vi "Scan Mode Panel.vi"(8 "error in (no error)":errorcluster, 11 "Scan SBlock in":refnum<class "Scan SBlock.lvclass">) -> (0 "error out":errorcluster, 2 "Parameters out":string[][][](array[string]), 3 "Schedule Block out":refnum<class "Schedule Block.lvclass">)   [LabVIEW 2020, in "TALOS.lvlib" / "Run Utilities.lvlib" / "Scan SBlock.lvclass"]
uses:
  Scan SBlock.lvclass
  Advanced Parameters.ctl
  Advanced Panel Parameter Mode.ctl
  Advanced Parameters - list.ctl
  Schedule Block/Schedule Block.lvclass
  C:/LabVIEW Code/TALOS/talos/Run Utilities/Schedule Block/Schedule Block.lvclass
panel:
  in  "Array from List":T1[](array[typedef]) caption="Parameters"
  in  "No. of steps":u32
  in  "Array of Parameters":T2[](array[typedef])
  # "Parameter"
  # "Values"
  # "If the LINKED mode is used the Step size is ignored, and it is calculated based on the number of steps -->"
  # "Parameter"
  # "From"
  # "To"
  # "Step"
  # "Mode"
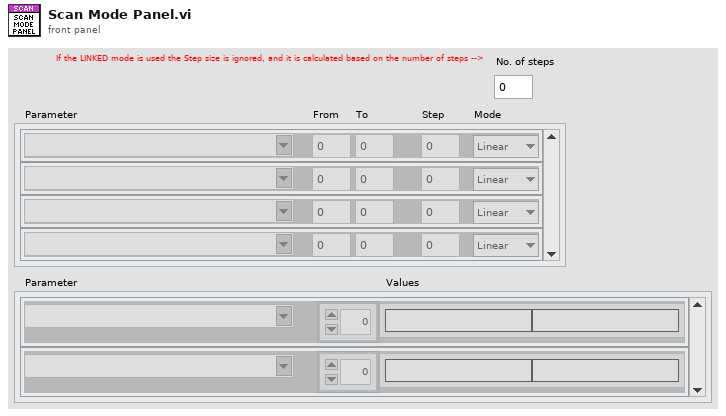
[diagram p1: front panel]
types:
  T1 = typedef "TALOS.lvlib/Run Utilities.lvlib/Scan SBlock.lvclass/Advanced Parameters - list.ctl" = cluster{"Param":string, "List of values":string[]}
  T2 = typedef "TALOS.lvlib/Run Utilities.lvlib/Scan SBlock.lvclass/Advanced Parameters.ctl" = cluster{"Param":string, "From":dbl, "To":dbl, "Step":dbl, "Mode":T3}
  T3 = typedef "TALOS.lvlib/Run Utilities.lvlib/Scan SBlock.lvclass/Advanced Panel Parameter Mode.ctl" = enum16{"Linear", "Log", "LINKED"}
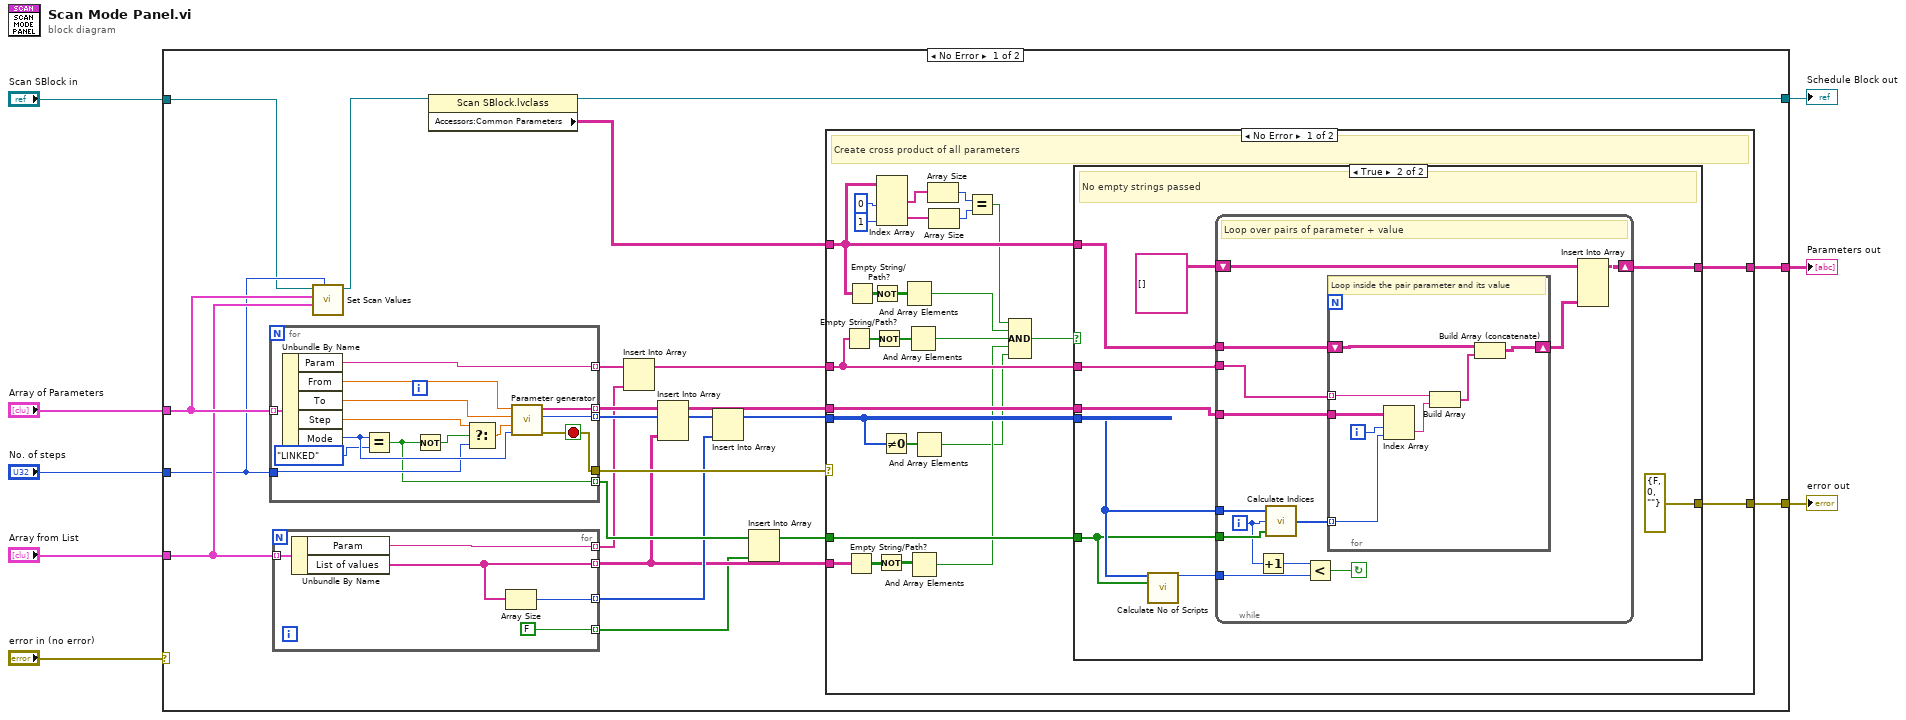
[diagram p0: block diagram]
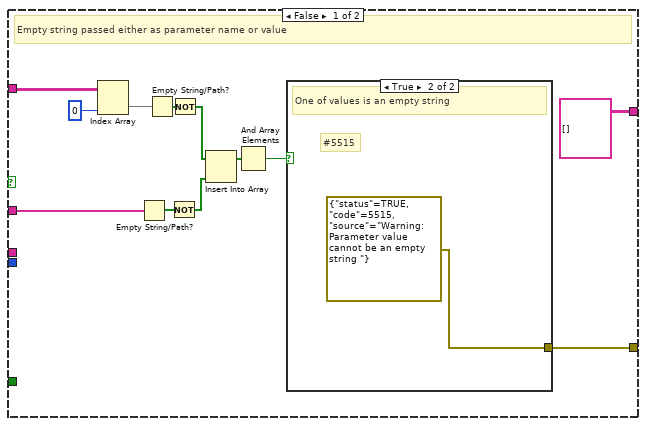
[diagram p2: hidden frame]
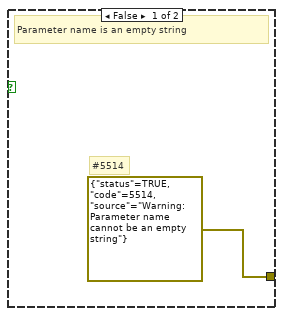
[diagram p3: hidden frame]
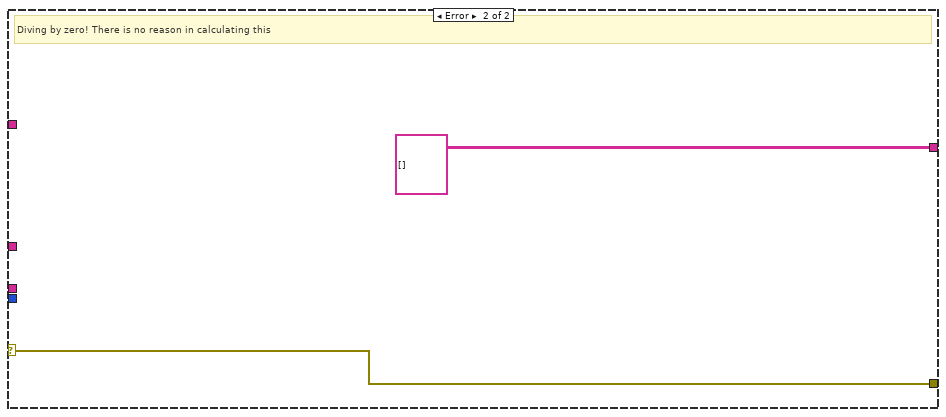
[diagram p4: hidden frame]
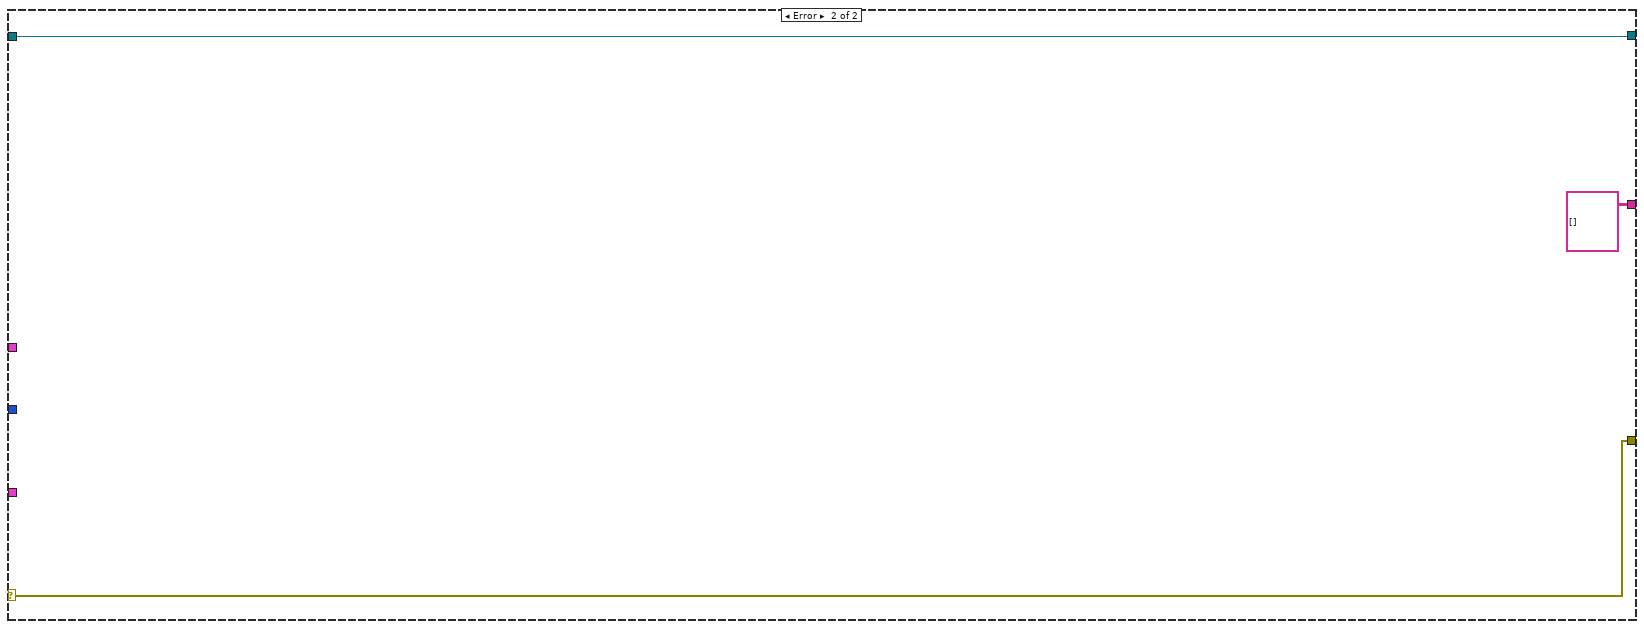
[diagram p5: hidden frame]
diagram:
  n1 = case shown="No Error" "error in (no error)" {
    selector: "error in (no error)" -> [_ w124]
    tunnel: [w29 string[][][] [] ("Parameters out")] -> w8
    tunnel: [w28 w124] -> w7
    tunnel: "Array of Parameters" -> [w15 _]
    tunnel: "Array from List" -> [w14 _]
    tunnel: "No. of steps" -> [w13 _]
    tunnel: "Scan SBlock in" -> [w12 w125]
    tunnel: [w9 w125] -> w2
    frame No Error {
      n2 = for {
        tunnel: w15 -> [w46] mode=indexing
        tunnel: w13 -> [w44]
        tunnel: [w42] -> w30
        tunnel: [w45] -> w24 mode=indexing
        tunnel: [w36] -> w26 mode=indexing
        tunnel: [w41] -> w27 mode=indexing
        tunnel: [w39] -> w25 mode=indexing
        stop <- w42 stop-if-true
        n3 = Unbundle By Name(w46) -> ("Param"=w45:string, "From"=w43:dbl, "To"=w47:dbl, "Step"=w48:dbl, "Mode"=w49:T3)
        n4 = Equal?(x=w49, y=Advanced_Panel_Parameter_Mode."LINKED") -> (x = y?=w36:bool)
        n5 = Not(x=w36) -> (.not. x?=w37:bool)
        n6 = Select(t=w48, s=w37, f=w44) -> (s? t:f=w40:dbl)
        n7 = call "Parameter generator.vi"("Mode"=w49, "Step/Iterations"=w40, "To"=w47, "From"=w43) -> ("error out"=w42:errorcluster, "Size of the array"=w41:i32, "Array of parameter values"=w39:string[])  [unwired: 5 in]
      }
      n8 = for {
        tunnel: w14 -> [w35] mode=indexing
        tunnel: [w34] -> w19 mode=indexing
        tunnel: [w33] -> w22 mode=indexing
        tunnel: [w32] -> w17 mode=indexing
        tunnel: [FALSE] -> w16 mode=indexing
        n9 = Unbundle By Name(w35) -> ("Param"=w33:string, "List of values"=w32:string[])
        n10 = Array Size(array=w32) -> (size(s)=w34:i32)
      }
      n11 = call-dynamic "Set Scan Values.vi"("No. of steps"=w13, "Array from List"=w14, "Array of Parameters"=w15, "Scan SBlock in"=w12) -> ("Scan SBlock out"=w10:refnum<class "Scan SBlock.lvclass">)  [unwired: 6 in, 1 out]
      n12 = property class="Scan SBlock.lvclass"(reference=w10) -> (reference out=w9:refnum<class "Scan SBlock.lvclass">, "Accessors:Common Parameters"=w11:string[][])  [unwired: 1 in, 1 out]
      n13 = Insert Into Array(array=w24, new element=w22) -> (w23:string[])  [unwired: 1 in]
      n14 = Insert Into Array(array=w25, new element=w17) -> (w21:string[][])  [unwired: 2 in]
      n15 = Insert Into Array(array=w27, new element=w19) -> (w20:i32[])  [unwired: 1 in]
      n16 = Insert Into Array(array=w26, new element=w16) -> (w18:bool[])  [unwired: 1 in]
      n17 = case shown="No Error" w30 {
        selector: w30 -> [_ w121]
        tunnel: [w75 string[][][] [] ("Parameters out")] -> w29
        tunnel: w21 -> [w72 _]
        tunnel: w11 -> [w59 _]
        tunnel: [w76 w121] -> w28
        tunnel: w23 -> [w73 _]
        tunnel: w20 -> [w55 _]
        tunnel: w18 -> [w74 _]
        tunnel: w17 -> [w50 _]
        frame No Error {
          # "Create cross product of all parameters"
          n18 = Empty String/Path?(string/path=w73) -> (empty?=w64:bool[])
          n19 = Empty String/Path?(string/path=w50) -> (empty?=w63:bool[][])
          n20 = Empty String/Path?(string/path=w59) -> (empty?=w67:bool[][])
          n21 = Not(x=w67) -> (.not. x?=w66:bool[][])
          n22 = Not(x=w64) -> (.not. x?=w65:bool[])
          n23 = Not(x=w63) -> (.not. x?=w62:bool[][])
          n24 = Index Array(array=w59, index (col) #1=0 ("disabled index (col)"), index (col) #2=1 ("index (col)")) -> (element #1=w58:string[], element #2=w61:string[])  [unwired: 2 in]
          n25 = Not Equal To 0?(x=w55) -> (x != 0?=w54:bool[])
          n26 = And Array Elements(Boolean array=w66) -> (logical AND=w71:bool)
          n27 = And Array Elements(Boolean array=w65) -> (logical AND=w69:bool)
          n28 = And Array Elements(Boolean array=w62) -> (logical AND=w70:bool)
          n29 = And Array Elements(Boolean array=w54) -> (logical AND=w53:bool)
          n30 = Array Size(array=w58) -> (size(s)=w57:i32)
          n31 = Array Size(array=w61) -> (size(s)=w60:i32)
          n32 = Equal?(x=w57, y=w60) -> (x = y?=w56:bool)
          n33 = Compound Arithmetic op=AND(w56, w71, w69, w70, w53) -> (w68:bool)
          n34 = case shown="True" w68 {
            tunnel: [w85 errorcluster {"status"=FALSE, "code"=0, "source"=""} ("error out")] -> w76
            tunnel: [string[][][] [] ("Parameters out") w97] -> w75
            tunnel: w55 -> [_ w95]
            tunnel: w74 -> [_ w94]
            tunnel: w59 -> [w88 w93]
            tunnel: w73 -> [w86 w92]
            tunnel: w72 -> [_ w91]
            frame False {
              # "Empty string passed either as parameter name or value"
              n35 = Index Array(array=w88, index (col)=0 ("disabled index (col)")) -> (element=w78:string[])  [unwired: 1 in]
              n36 = Empty String/Path?(string/path=w86) -> (empty?=w82:bool[])
              n37 = Empty String/Path?(string/path=w78) -> (empty?=w83:bool[])
              n38 = Not(x=w82) -> (.not. x?=w80:bool[])
              n39 = Not(x=w83) -> (.not. x?=w81:bool[])
              n40 = Insert Into Array(array=w81, new element=w80) -> (w79:bool[])  [unwired: 1 in]
              n41 = And Array Elements(Boolean array=w79) -> (logical AND=w77:bool)
              n42 = case shown="True" w77 {
                tunnel: [errorcluster {"status"=TRUE, "code"=5514, "source"="Warning: Parameter name cannot be an empty string"} ("error out") errorcluster {"status"=TRUE, "code"=5515, "source"="Warning: Parameter value cannot be an empty string "} ("error out")] -> w85
                frame False {
                  # "#5514"
                  # "Parameter name is an empty string"
                }
                frame True {
                  # "#5515"
                  # "One of values is an empty string"
                }
              }
            }
            frame True {
              # "No empty strings passed"
              n43 = call "Calculate No of Scripts.vi"("Sizes of Arrays"=w95, "Linked? Array"=w94) -> ("No of scripts"=w96:i32)  [unwired: 13 in]
              n44 = while {
                shift-right: [w110] -> w97
                shift-left: string[][][] [] ("Parameters out") -> [w109]
                tunnel: w92 -> [w112]
                tunnel: w93 -> [w108]
                tunnel: w91 -> [w111]
                tunnel: w96 -> [w102]
                tunnel: w95 -> [w104]
                tunnel: w94 -> [w103]
                i -> [w101]
                stop <- w106 continue-if-true
                # "Loop over pairs of parameter + value"
                n45 = Increment(x=w101) -> (x+1=w100:i32)
                n46 = call "Calculate Indices.vi"("Linked? Array"=w103, "Index of script"=w101, "Sizes of Arrays"=w104) -> ("Indices"=w105:i32[])
                n47 = Less?(x=w100, y=w102) -> (x < y?=w106:bool)
                n48 = for {
                  tunnel: w112 -> [w115] mode=indexing
                  tunnel: w111 -> [w116]
                  shift-right: [w119] -> w107
                  shift-left: w108 -> [w118]
                  tunnel: w105 -> [w117] mode=indexing
                  i -> [w120]
                  # "Loop inside the pair parameter and its value"
                  n49 = Index Array(array=w116, index (row)=w120, index (col)=w117) -> (element=w113:string)
                  n50 = Build Array(w115, w113) -> (w114:string[])
                  n51 = Build Array (concatenate)(w118, w114) -> (w119:string[][])
                }
                n52 = Insert Into Array(array=w109, new element=w107) -> (w110:string[][][])  [unwired: 3 in]
              }
            }
          }
        }
        frame Error {
          # "Diving by zero! There is no reason in calculating this"
        }
      }
    }
    frame Error {
    }
  }
  "Parameters out" <- w8
  "error out" <- w7
  "Schedule Block out" <- w2
